vi "testCan.vi"() -> ()   [LabVIEW 2014]
uses:
  <vilib>/CANopenLib/CANOPEN.llb/CANopen BaudRate.ctl
  <vilib>/CANopenLib/CANOPEN.llb/CANopen Interface Create.vi
  <vilib>/CANopenLib/CANOPEN.llb/CANopen CAN Frame Read Create.vi
panel:
  out "Fehler (Ausgang)":errorcluster
  out "Tabellenelement":string[][](table)=[["10", "23"]]
  in  "Stopp":bool
  in  "baud rate":T1=2 items=["1 Mbit/s"=0, "800 kbit/s"=1, "500 kbit/s"=2, "250 kbit/s"=3, "125 kbit/s"=4, "50 kbit/s"=6, "20 kbit/s"=7, "10 kbit/s"=8]
  in  "interface name":u32(ring) items=["CANopen01", "CANopen02", "CANopen03", "CANopen04", "CANopen05", "CANopen06", "CANopen07", "CANopen08", "CANopen09", "CANopen10", "CANopen11", "CANopen12", "CANopen13", "CANopen14", "CANopen15", "CANopen16", "CANopen17", "CANopen18", "CANopen19", "CANopen20", "CANopen21", "CANopen22", "CANopen23", "CANopen24", "CANopen25", "CANopen26", "CANopen27", "CANopen28", "CANopen29", "CANopen30", "CANopen31", "CANopen32"]
  # "Empfängt Daten. COB-ID und Daten in Hex-Form werden in der Tabelle abelegt."
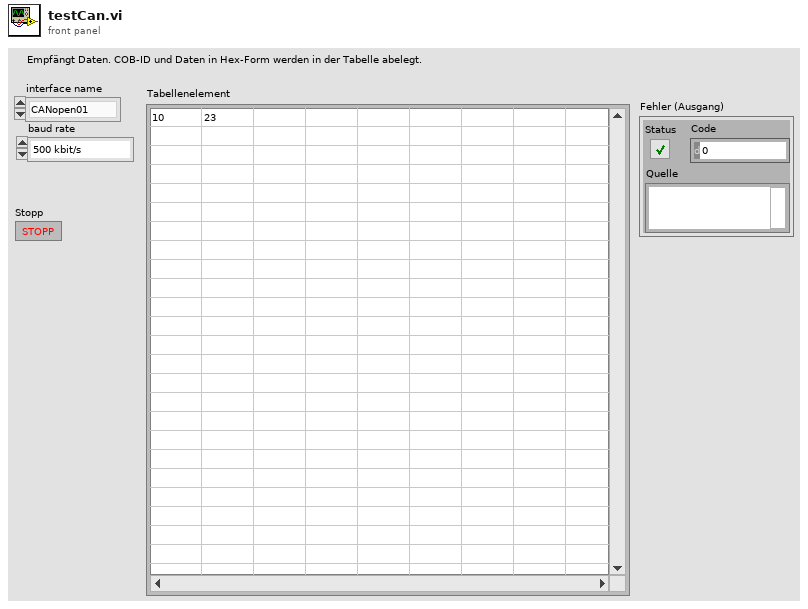
[diagram p1: front panel]
types:
  T1 = typedef "CANopen BaudRate.ctl" = u32
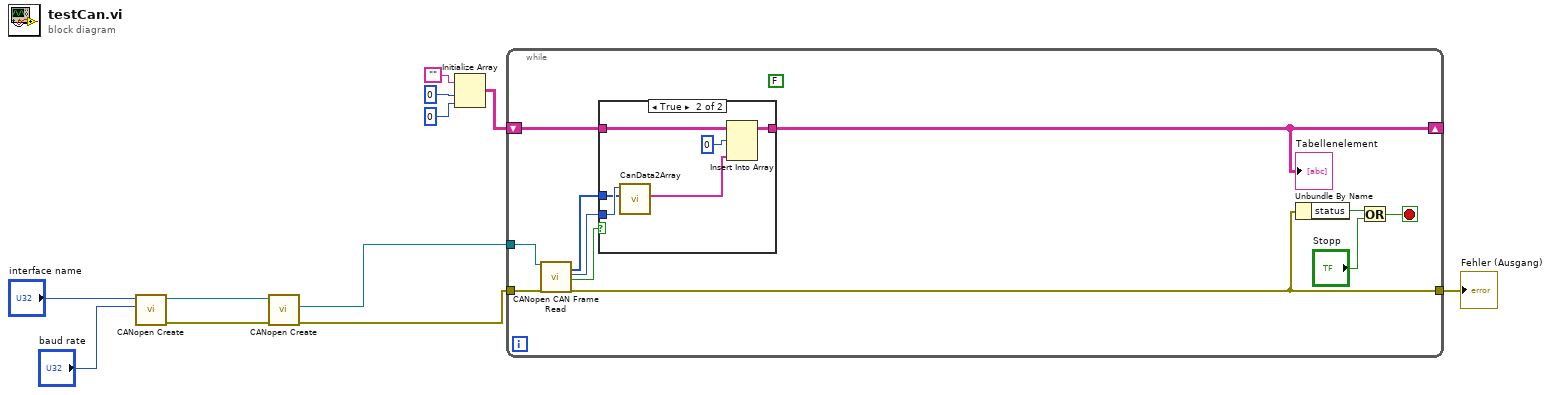
[diagram p0: block diagram]
diagram:
  n1 = call-poly <vilib>:"CANopen Create.vi"("baud rate"="baud rate", "interface name"="interface name") -> ("error out"=w8:errorcluster, "interface object out"=w9:refnum<k20>)  [unwired: 8 in]
  n2 = call-poly <vilib>:"CANopen Create.vi"("error in (no error)"=w8, "interface object in"=w9) -> ("error out"=w1:errorcluster, "CAN frame read object out"=w7:refnum<k20>)  [unwired: 7 in, 1 out]
  n3 = Initialize Array("" ("Element"), 0 ("Dimension"), 0 ("Dimension")) -> (w3:string[][])
  n4 = while {
    tunnel: w7 -> [w22]
    tunnel: w1 -> [w21]
    shift-right: [w13] -> _
    shift-left: w3 -> [w16]
    tunnel: [w12] -> w2
    stop <- w20 stop-if-true
    (unwired) FALSE
    n5 = call <vilib>:"CANopen CAN Frame Read.vi"("CAN frame read object in"=w22, "error in (no error)"=w21) -> ("CAN message data"=w14:u8[], "COB-ID"=w15:u32, "new data?"=w17:bool, "error out"=w12:errorcluster)  [unwired: 11 in, 3 out]
    n6 = case shown="True" w17 {
      tunnel: w16 -> [w23 w28]
      tunnel: w15 -> [_ w27]
      tunnel: w14 -> [_ w26]
      tunnel: [w23 w25] -> w13
      frame False {
      }
      frame True {
        n7 = call "CanData2Array.vi"("Data"=w26, "COB ID"=w27) -> ("Array"=w24:string[])  [unwired: 9 in]
        n8 = Insert Into Array(array=w28, index (row)=0 ("Index (Zeile)"), new element=w24) -> (w25:string[][])  [unwired: 1 in]
      }
    }
    "Tabellenelement" <- w13
    n9 = Unbundle By Name(w12) -> ("status"=w18:bool)
    n10 = Or(x=w18, y="Stopp") -> (x .or. y?=w20:bool)
  }
  "Fehler (Ausgang)" <- w2
